vi "CreateProduct.vi"(8 "Error In":errorcluster, 11 "reference in":refnum<class "HatchbackCarFactory.lvclass">) -> (0 "Error Out":errorcluster, 2 "ICarProduct":refnum<class "ICarProduct.lvclass">, 3 "reference out":refnum<class "HatchbackCarFactory.lvclass">)   [LabVIEW 2024, in "HatchbackCarFactory.lvclass"]
uses:
  HatchbackCarFactory.lvclass
  HatchbackCarFactory.lvclass/HatchbackCarFactory.ctl
  Hatchback/Hatchback.lvclass
  C:/Users/burakkorkmaz/Desktop/Leveling/labview-design-patterns/Factory Method Pattern/Labview/Hatchback/Hatchback.lvclass
  C:/Users/burakkorkmaz/Desktop/Leveling/labview-design-patterns/Factory Method Pattern/Labview/ICarProduct/ICarProduct.lvclass
  ICarProduct/ICarProduct.lvclass
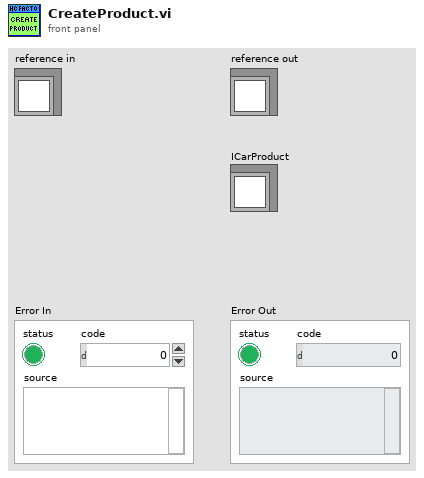
[diagram p1: front panel]
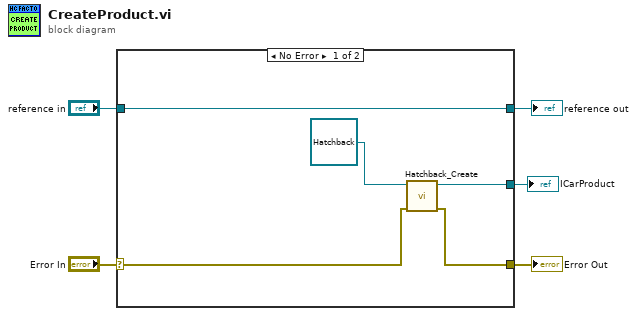
[diagram p0: block diagram]
diagram:
  n1 = case shown="No Error" "Error In" {
    selector: "Error In" -> [w7 w12]
    tunnel: [w6 w12] -> w4
    tunnel: [w10 w11] -> w2
    tunnel: "reference in" -> [w10 w11]
    tunnel: [w9 _] -> w1
    frame No Error {
      n2 = call "Hatchback_Create.vi"("Error In"=w7, "reference in"=refnum<class "Hatchback.lvclass"> refnum ("Hatchback")) -> ("Error Out"=w6:errorcluster, "reference out"=w9:refnum<class "Hatchback.lvclass">)  [unwired: 8 in]
    }
    frame Error {
    }
  }
  "Error Out" <- w4
  "reference out" <- w2
  "ICarProduct" <- w1
